vi "CH3_Comm_TCPIP.vi"() -> ()   [LabVIEW 2018]
uses:
  TCPIP/TCPIP.lvclass
  RxTx/RxTx.lvclass
panel:
  out "error out":errorcluster
  in  "Channel:":u16=3
  in  "RxTx.lvclass":refnum<class "RxTx.lvclass">
  in  "TCPIP.lvclass":refnum<class "TCPIP.lvclass">
  in  "remote port":u16=59003
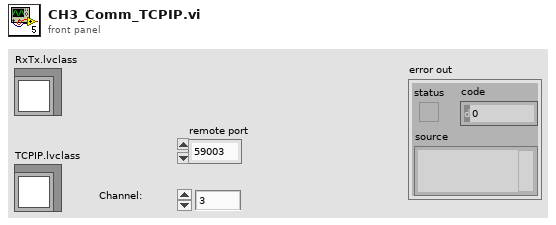
[diagram p1: front panel]
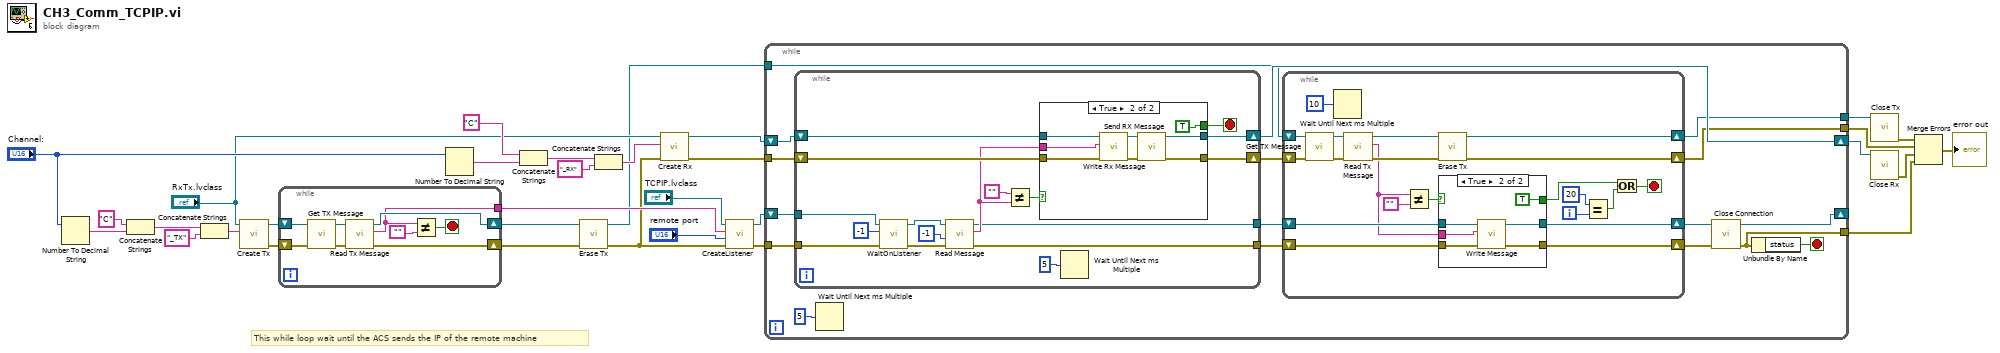
[diagram p0: block diagram]
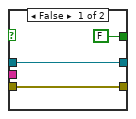
[diagram p2: hidden frame]
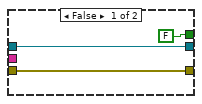
[diagram p3: hidden frame]
diagram:
  # "This while loop wait until the ACS sends the IP of the remote machine"
  n1 = Number To Decimal String(number="Channel:") -> (decimal integer string=w29:string)  [unwired: 1 in]
  n2 = Concatenate Strings("C", w29) -> (w26:string)
  n3 = Concatenate Strings(w26, "_TX" ("Reader Name")) -> (w27:string)
  n4 = call "Create Tx.vi"("Writer Name"=w27, "RxTx in"="RxTx.lvclass") -> ("error out"=w6:errorcluster, "RxTx out"=w7:refnum<class "RxTx.lvclass">)  [unwired: 8 in]
  n5 = while {
    shift-right: [w38] -> w4
    shift-left: w6 -> [w36]
    shift-right: [w39] -> w1
    shift-left: w7 -> [w41]
    tunnel: [w33] -> w5
    stop <- w34 stop-if-true
    n6 = call "Get TX Message.vi"("error in (no error)"=w36, "RxTx in"=w41) -> ("error out"=w37:errorcluster, "RxTx out"=w40:refnum<class "RxTx.lvclass">)  [unwired: 8 in]
    n7 = call "Read Tx Message.vi"("error in (no error)"=w37, "RxTx in"=w40) -> ("error out"=w38:errorcluster, "Tx Message"=w33:string, "RxTx out"=w39:refnum<class "RxTx.lvclass">)  [unwired: 7 in]
    n8 = Not Equal?(x=w33, y="") -> (x != y?=w34:bool)
  }
  n9 = Number To Decimal String(number="Channel:") -> (decimal integer string=w23:string)  [unwired: 1 in]
  n10 = Concatenate Strings("C", w23) -> (w21:string)
  n11 = call "Erase Tx.vi"("error in (no error)"=w4, "RxTx in"=w1) -> ("error out"=w3:errorcluster, "RxTx out"=w2:refnum<class "RxTx.lvclass">)  [unwired: 8 in]
  n12 = Concatenate Strings(w21, "_RX" ("Reader Name")) -> (w19:string)
  n13 = call "Create Rx.vi"("error in (no error)"=w3, "Reader Name"=w19, "RxTx in"="RxTx.lvclass") -> ("error out"=w24:errorcluster, "RxTx out"=w16:refnum<class "RxTx.lvclass">)  [unwired: 7 in]
  n14 = call-dynamic "CreateListener.vi"("error in (no error)"=w3, "remote port"="remote port", "IP"=w5, "TCPIP in"="TCPIP.lvclass") -> ("error out"=w30:errorcluster, "TCPIP out"=w13:refnum<class "TCPIP.lvclass">)  [unwired: 6 in]
  n15 = while {
    tunnel: w30 -> [w58]
    tunnel: w24 -> [w57]
    tunnel: w2 -> [w43]
    shift-right: [w54] -> w15
    shift-left: w16 -> [w55]
    tunnel: [w53] -> w14
    tunnel: [w52] -> w12
    tunnel: [w45] -> w9
    shift-right: [w47] -> _
    shift-left: w13 -> [w46]
    stop <- w44 stop-if-true
    n16 = while {
      shift-right: [w93] -> w42
      shift-left: w57 -> [w105]
      shift-right: [w94] -> w54
      shift-left: w55 -> [w104]
      tunnel: w46 -> [w98]
      tunnel: w58 -> [w97]
      tunnel: [w91] -> w51
      tunnel: [w90] -> w50
      stop <- w92 stop-if-true
      n17 = call-dynamic "WaitOnListener.vi"("error in (no error)"=w97, "timeout ms"=-1, "TCPIP in"=w98) -> ("error out"=w95:errorcluster, "TCPIP out"=w96:refnum<class "TCPIP.lvclass">)  [unwired: 7 in]
      n18 = call "Read Message.vi"("error in (no error)"=w95, "timeout"=-1, "TCPIP in"=w96) -> ("error out"=w90:errorcluster, "Message"=w100:string, "TCPIP out"=w91:refnum<class "TCPIP.lvclass">)  [unwired: 6 in]
      n19 = Not Equal?(x="", y=w100) -> (x != y?=w102:bool)
      n20 = case shown="True" w102 {
        tunnel: w105 -> [w107 w114]
        tunnel: w104 -> [w108 w113]
        tunnel: [w108 w111] -> w94
        tunnel: [w107 w110] -> w93
        tunnel: w100 -> [_ w112]
        tunnel: [FALSE TRUE] -> w92
        frame False {
        }
        frame True {
          n21 = call "Write Rx Message.vi"("error in (no error)"=w114, "Rx Message"=w112, "RxTx in"=w113) -> ("error out"=w115:errorcluster, "RxTx out"=w116:refnum<class "RxTx.lvclass">)  [unwired: 7 in]
          n22 = call "Send RX Message.vi"("error in (no error)"=w115, "RxTx in"=w116) -> ("error out"=w110:errorcluster, "RxTx out"=w111:refnum<class "RxTx.lvclass">)  [unwired: 8 in]
        }
      }
      n23 = Wait Until Next ms Multiple(millisecond multiple=u32 5) -> ()  [unwired: 1 out]
    }
    n24 = Wait Until Next ms Multiple(millisecond multiple=u32 5) -> ()  [unwired: 1 out]
    n25 = while {
      shift-right: [w68] -> w49
      shift-left: w51 -> [w77]
      shift-right: [w67] -> w48
      shift-left: w50 -> [w76]
      shift-right: [w79] -> w53
      shift-left: w43 -> [w66]
      shift-right: [w78] -> w52
      shift-left: w42 -> [w65]
      i -> [w63]
      stop <- w59 stop-if-true
      n26 = call "Get TX Message.vi"("error in (no error)"=w65, "RxTx in"=w66) -> ("error out"=w75:errorcluster, "RxTx out"=w71:refnum<class "RxTx.lvclass">)  [unwired: 8 in]
      n27 = Wait Until Next ms Multiple(millisecond multiple=u32 10) -> ()  [unwired: 1 out]
      n28 = call "Read Tx Message.vi"("error in (no error)"=w75, "RxTx in"=w71) -> ("error out"=w72:errorcluster, "Tx Message"=w70:string, "RxTx out"=w73:refnum<class "RxTx.lvclass">)  [unwired: 7 in]
      n29 = Not Equal?(x=w70, y="") -> (x != y?=w69:bool)
      n30 = call "Erase Tx.vi"("error in (no error)"=w72, "RxTx in"=w73) -> ("error out"=w78:errorcluster, "RxTx out"=w79:refnum<class "RxTx.lvclass">)  [unwired: 8 in]
      n31 = case shown="True" w69 {
        tunnel: w70 -> [_ w88]
        tunnel: w77 -> [w82 w87]
        tunnel: w76 -> [w81 w86]
        tunnel: [w82 w85] -> w68
        tunnel: [w81 w84] -> w67
        tunnel: [FALSE TRUE] -> w61
        frame False {
        }
        frame True {
          n32 = call "Write Message.vi"("error in (no error)"=w86, "Message"=w88, "TCPIP in"=w87) -> ("error out"=w84:errorcluster, "TCPIP out"=w85:refnum<class "TCPIP.lvclass">)  [unwired: 7 in]
        }
      }
      n33 = Equal?(x=20, y=w63) -> (x = y?=w60:bool)
      n34 = Or(x=w61, y=w60) -> (x .or. y?=w59:bool)
    }
    n35 = call "Close Connection.vi"("error in (no error)"=w48, "TCPIP in"=w49) -> ("error out"=w45:errorcluster, "TCPIP out"=w47:refnum<class "TCPIP.lvclass">)  [unwired: 8 in]
    n36 = Unbundle By Name(w45) -> ("status"=w44:bool)
  }
  n37 = call "Close Tx.vi"("RxTx in"=w14) -> ("error out"=w10:errorcluster)  [unwired: 9 in, 1 out]
  n38 = call "Close Rx.vi"("RxTx in"=w15) -> ("error out"=w8:errorcluster)  [unwired: 9 in, 1 out]
  n39 = Merge Errors(w10, w12, w8, w9) -> (→"error out":errorcluster)
